vi "_Serial_Mark10-Config (Moving Speed).vi"(4 "Speed(mm/min)":dbl, 5 "Serial Port":refnum<visa-resource-name>="COM5") -> (2 "VISA resource name out":refnum<visa-resource-name>)   [LabVIEW 2015]
panel:
  out "TX String":string
  # "MARK10 Set moving speed"
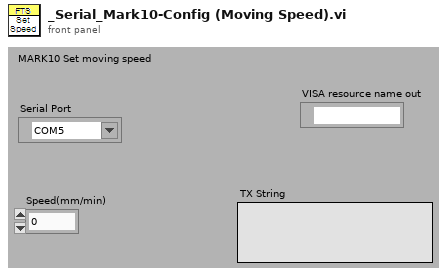
[diagram p1: front panel]
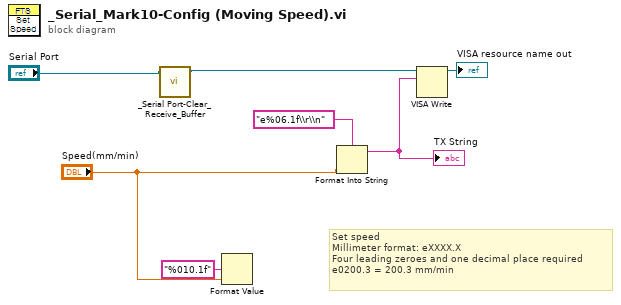
[diagram p0: block diagram]
diagram:
  # "Set speed\nMillimeter format: eXXXX.X\nFour leading zeroes and one decimal place required\ne0200.3 = 200.3 mm/min"
  n1 = call "_Serial Port-Clear_Receive_Buffer.vi"("Serial Port"="Serial Port") -> ("Serial Port out"=w1:refnum<visa-resource-name>)  [unwired: 3 in, 1 out]
  n2 = Format Value(format string="%010.1f" ("포맷 문자열"), value (0)="Speed(mm/min)") -> ()  [unwired: 1 in, 1 out]
  n3 = Format Into String(format string="e%06.1f\\r\\n" ("포맷 문자열"), "Speed(mm/min)") -> (resulting string=w6:string)  [unwired: 2 in, 1 out]
  "TX String" <- w6
  n4 = VISA Write(VISA resource name=w1, write buffer=w6) -> (VISA resource name out=→"VISA resource name out":refnum<visa-resource-name>)  [unwired: 1 in, 2 out]
